vi "Update GUI for Config Local Daq.vi"(6 "Voltage Ring":refnum<vi>, 8 "error in (no error)":errorcluster, 9 "Digital in":refnum<vi>, 10 "Ring Refnum":refnum<vi>, 11 "Clust Refnum 2":refnum<vi>) -> (0 "error out":errorcluster, 1 "AI.Voltage.Rngs":dbl[](array[numeric]), 2 "AI.MaxMultiChanRate":dbl, 3 "Channels":string, 4 "Port locations":string[](array[string]))   [LabVIEW 2019]
uses:
  Local Daq Config.ctl
  <resource>/objmgr/daqmx.rc
panel:
  out "Number of Channels":dbl
  out "Voltage":dbl[](array[numeric])
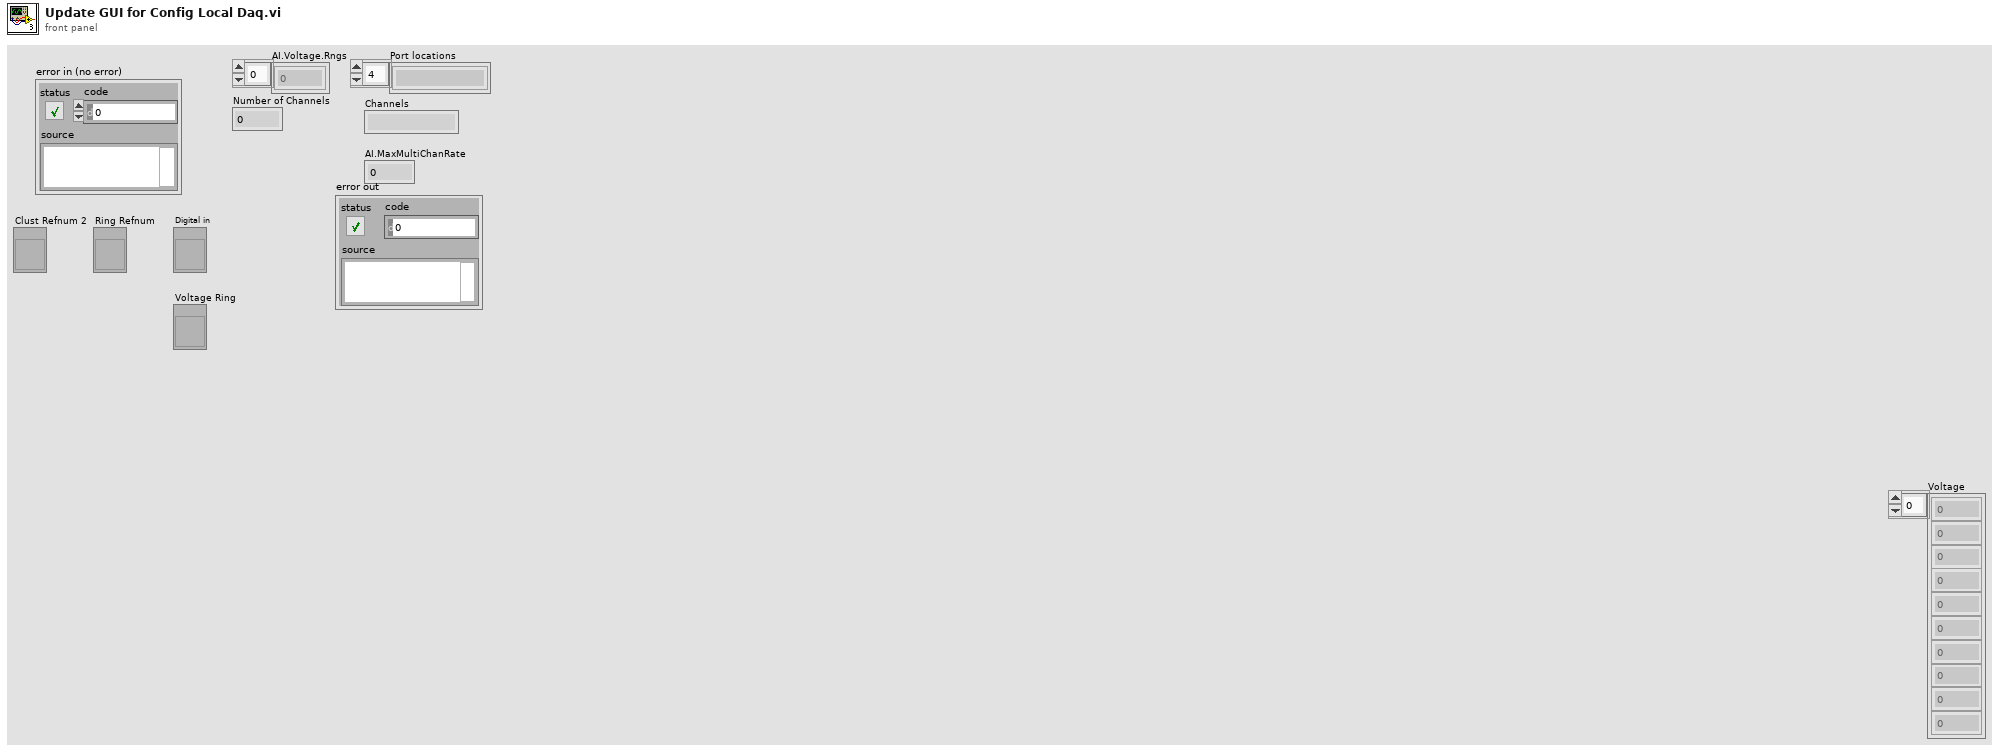
[diagram p1: front panel]
types:
  T1 = typedef "Local Daq Config.ctl" = cluster{"Sample rate (Hz)":dbl, "Over sample factor":dbl, "Terminal Configuration":enum16{"Single Ended", "Differential"}, "Device":u16, "Max Voltage":u16}
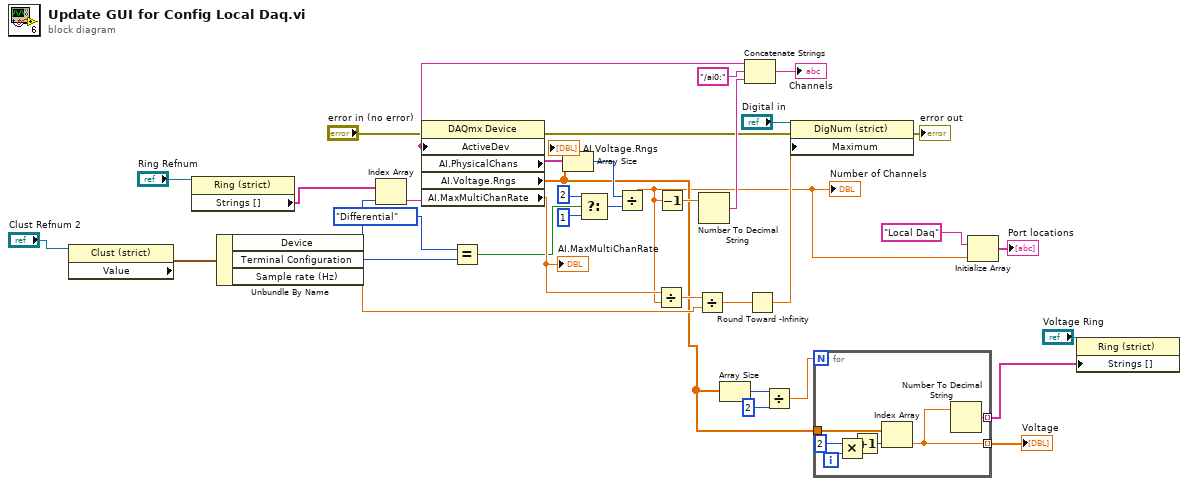
[diagram p0: block diagram]
diagram:
  n1 = property class="Clust (strict)"(reference="Clust Refnum 2") -> ("Value"=w14:T1)  [unwired: 1 in, 2 out]
  n2 = property class="Ring (strict)"(reference="Ring Refnum") -> ("Strings []"=w12:string[])  [unwired: 1 in, 2 out]
  n3 = Unbundle By Name(w14) -> ("Device"=w19:u16, "Terminal Configuration"=w37:enum16{"Single Ended", "Differential"}, "Sample rate (Hz)"=w35:dbl)
  n4 = Index Array(array=w12, index=w19) -> (element=w18:string)
  n5 = property class="DAQmx Device"(error in="error in (no error)", "ActiveDev"=w18) -> (error out=w16:errorcluster, "AI.PhysicalChans"=w29:tag[], "AI.Voltage.Rngs"=w7:dbl[], "AI.MaxMultiChanRate"=w30:dbl)  [unwired: 1 in, 1 out]
  "AI.MaxMultiChanRate" <- w30
  "AI.Voltage.Rngs" <- w7
  n6 = Equal?(x=enum16{"Single Ended", "Differential"}."Differential" ("Terminal Configuration"), y=w37) -> (x = y?=w25:bool)
  n7 = Array Size(array=w29) -> (size(s)=w31:i32)
  n8 = Select(t=2, s=w25, f=1) -> (s? t:f=w28:i32)
  n9 = Divide(x=w31, y=w28) -> (x/y=w3:dbl)
  "Number of Channels" <- w3
  n10 = Divide(x=w30, y=w3) -> (x/y=w32:dbl)
  n11 = Decrement(x=w3) -> (x-1=w22:dbl)
  n12 = Divide(x=w32, y=w35) -> (x/y=w33:dbl)
  n13 = Number To Decimal String(number=w22) -> (decimal integer string=w23:string)  [unwired: 1 in]
  n14 = Array Size(array=w7) -> (size(s)=w11:i32)
  n15 = Concatenate Strings(w18, "/ai0:" ("string"), w23) -> (→"Channels":string)
  n16 = Round Toward -Infinity(1:w33) -> (0:w34:dbl)
  n17 = Divide(x=w11, y=2) -> (x/y=w9:dbl)
  n18 = property on="Property Node" class="DigNum (strict)"(reference="Digital in", error in=w16, "Maximum"=w34) -> (error out=→"error out":errorcluster)  [unwired: 1 out]
  n19 = for {
    N: w9 -> [_]
    tunnel: w7 -> [w44]
    tunnel: [w39] -> w8 mode=indexing
    tunnel: [w38] -> w4 mode=indexing
    i -> [w42]
    n20 = Multiply(x=2, y=w42) -> (x*y=w43:i32)
    n21 = Increment(x=w43) -> (x+1=w40:i32)
    n22 = Index Array(array=w44, index=w40) -> (element=w39:dbl)
    n23 = Number To Decimal String(number=w39) -> (decimal integer string=w38:string)  [unwired: 1 in]
  }
  "Voltage" <- w8
  n24 = Initialize Array("Local Daq", w3) -> (→"Port locations":string[])
  n25 = property class="Ring (strict)"(reference="Voltage Ring", "Strings []"=w4) -> ()  [unwired: 1 in, 2 out]
